vi "Compare Match Pattern.vi"(4 "use cached delimeter pattern data? (F)":bool, 6 "delimeters":cluster{"start":string, "end":string}={"start"="{{", "end"="}}"}, 7 "ignore case? (F)":bool, 8 "error in (no error)":errorcluster, 9 "substitutions":map{string, string}(c390), 11 "string to match":string) -> (0 "error out":errorcluster, 3 "match?":bool)   [LabVIEW 2019]
doc: "<b>Description</b> This VI applies compares a templated reference string against a map of replacements. Non-templated elements in the input string are ignored.\n\nFor example, if the string to match is \"{{Foo:bar}} {{Biz:BAZ}}\" and the map contains the definitions {Foo => bar, Biz: baz} and the ignore case input were TRUE, this VI would output match = TRUE.\n\n<b>Inputs</b>\n<b>substitutions</b>: A dictoinary of substitutions to apply to the input string.\n<b>delimeters</b>: The start and end delimeters for the desired substitution pattern. Defaults to '{{' and '}}'.\n<b>string to match</b>: A string containing substituions to match.\n\n<b>Outputs</b>\n<b>error out</b>: This VI will return error -1967345147 if a substitution key is missing from the input dictionary.\n<b>match?</b>: True if the template expression matches the contents of the map.\n\nBSD 3-Clause License\n\nCopyright (c) 2021, TauTerra, LLC\nAll rights reserved.\n\nRedistribution and use in source and binary forms, with or without\nmodification, are permitted provided that the following conditions are met:\n\n1. Redistributions of source code must retain the above copyright notice, this\n list of conditions and the following disclaimer.\n\n2. Redistributions in binary form must reproduce the above copyright notice,\n this list of conditions and the following disclaimer in the documentation\n and/or other materials provided with the distribution.\n\n3. Neither the name of the copyright holder nor the names of its\n contributors may be used to endorse or promote products derived from\n this software without specific prior written permission.\n\nTHIS SOFTWARE IS PROVIDED BY THE COPYRIGHT HOLDERS AND CONTRIBUTORS \"AS IS\"\nAND ANY EXPRESS OR IMPLIED WARRANTIES, INCLUDING, BUT NOT LIMITED TO, THE\nIMPLIED WARRANTIES OF MERCHANTABILITY AND FITNESS FOR A PARTICULAR PURPOSE ARE\nDISCLAIMED. IN NO EVENT SHALL THE COPYRIGHT HOLDER OR CONTRIBUTORS BE LIABLE\nFOR ANY DIRECT, INDIRECT, INCIDENTAL, SPECIAL, EXEMPLARY, OR CONSEQUENTIAL\nDAMAGES (INCLUDING, BUT NOT LIMITED TO, PROCUREMENT OF SUBSTITUTE GOODS OR\nSERVICES; LOSS OF USE, DATA, OR PROFITS; OR BUSINESS INTERRUPTION) HOWEVER\nCAUSED AND ON ANY THEORY OF LIABILITY, WHETHER IN CONTRACT, STRICT LIABILITY,\nOR TORT (INCLUDING NEGLIGENCE OR OTHERWISE) ARISING IN ANY WAY OUT OF THE USE\nOF THIS SOFTWARE, EVEN IF ADVISED OF THE POSSIBILITY OF SUCH DAMAGE."
uses:
  6811bf61-4d49-4179-8fc7-a72229c4be46.vi
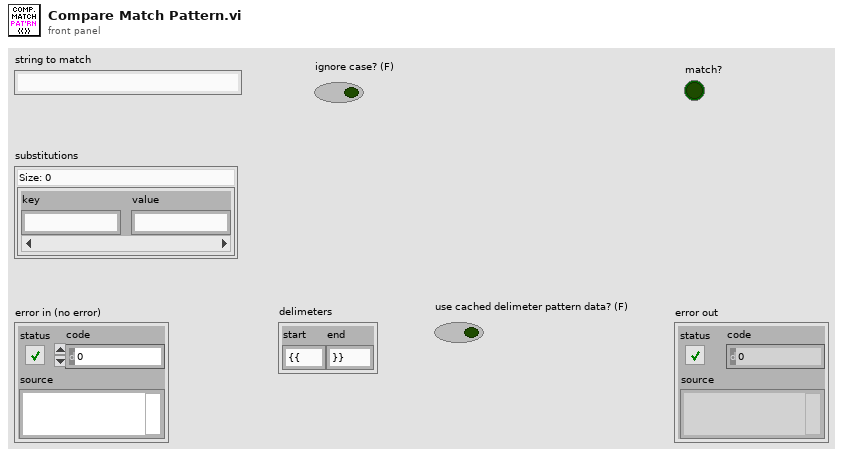
[diagram p1: front panel]
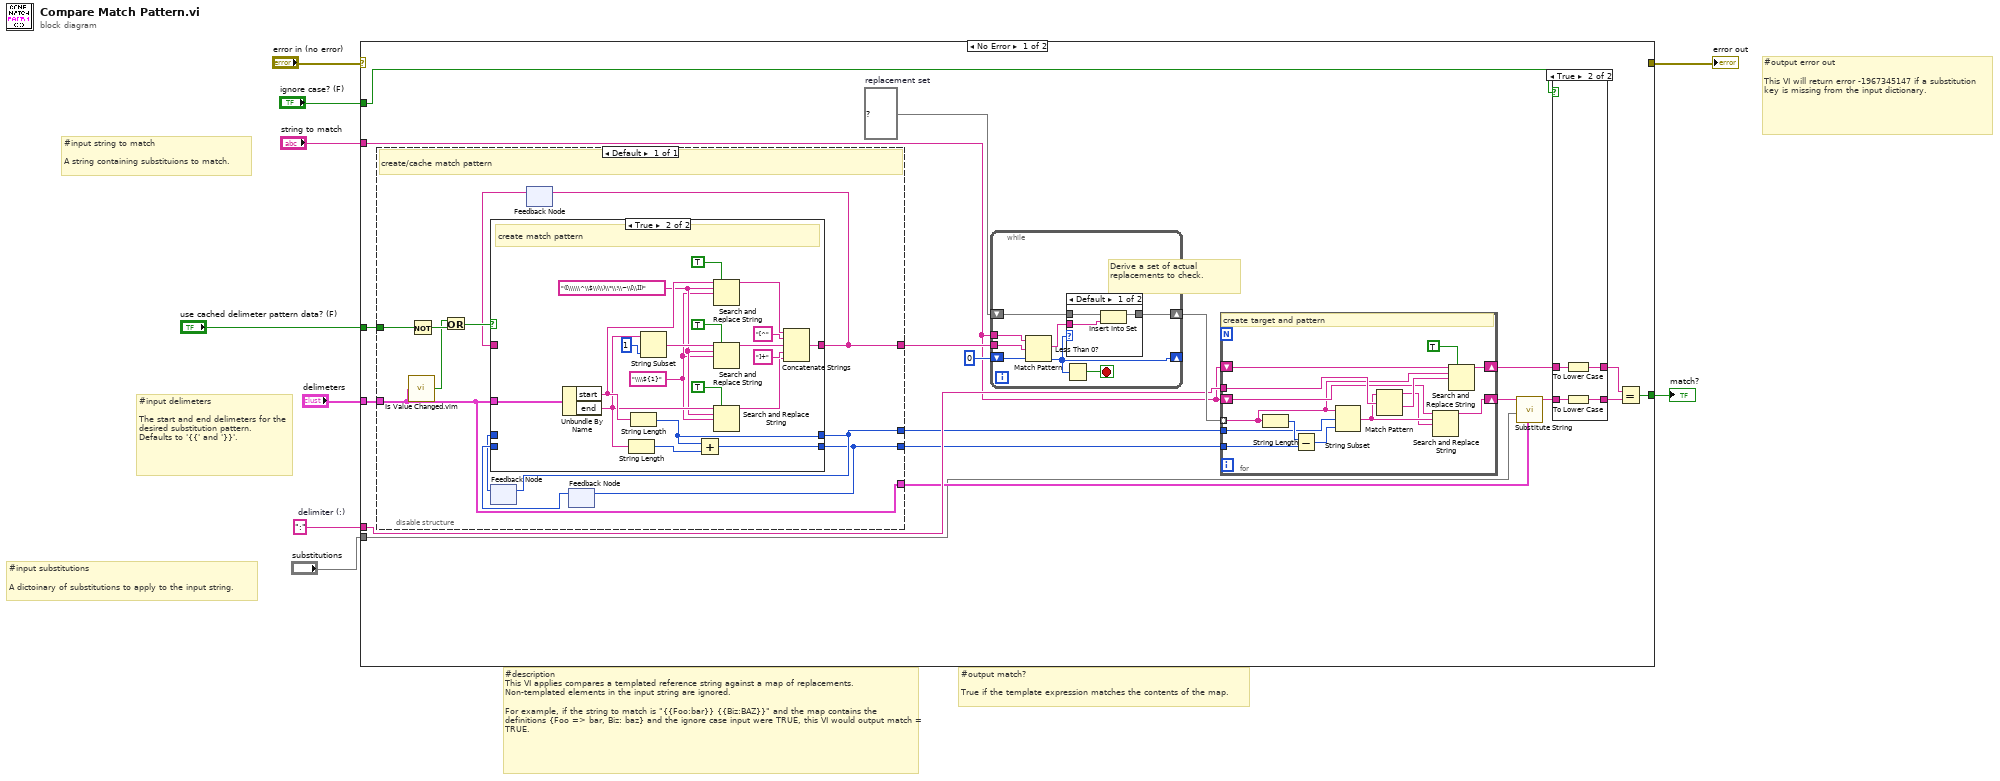
[diagram p0: block diagram]
diagram:
  w3 = ":"  # delimiter (:)
  # "#output error out\n\nThis VI will return error -1967345147 if a substitution key is missing from the input dictionary."
  # "#output match?\n\nTrue if the template expression matches the contents of the map."
  # "#input substitutions\n\nA dictoinary of substitutions to apply to the input string."
  # "#input delimeters\n\nThe start and end delimeters for the desired substitution pattern. Defaults to '{{' and '}}'."
  # "#input string to match\n\nA string containing substituions to match."
  # "#description\nThis VI applies compares a templated reference string against a map of replacements. Non-templated elements in the input string are ignored.\n\nFor example, if the string to match is \"{{Foo:bar}} {{Biz:BAZ}}\" and the map contains the definitions {Foo => bar, Biz: baz} and the ignore case input were TRUE, this VI would output match = TRUE."
  n1 = case shown="No Error" "error in (no error)" {
    selector: "error in (no error)" -> [_ w94]
    tunnel: "delimeters" -> [w26 _]
    tunnel: "string to match" -> [w19 _]
    tunnel: "substitutions" -> [w17 _]
    tunnel: [_ w94] -> w5
    tunnel: "use cached delimeter pattern data? (F)" -> [w25 _]
    tunnel: w3 -> [w22 _]
    tunnel: [w16 _] -> w2
    tunnel: "ignore case? (F)" -> [w15 _]
    frame No Error {
      w28 = set{string} {}  # replacement set
      n2 = disable-structure shown="Default" {
        disable-tunnel: w26 -> [w49]
        disable-tunnel: w25 -> [w59]
        disable-tunnel: [w55] -> w20
        disable-tunnel: [w54] -> w24
        disable-tunnel: [w53] -> w21
        disable-tunnel: [w49] -> w18
        frame Enabled {
          # "create/cache match pattern"
          n3 = call "Is Value Changed.vim"("value"=w49) -> ("changed or first call?"=w57:bool)
          n4 = Not(x=w59) -> (.not. x?=w58:bool)
          n5 = Or(x=w57, y=w58) -> (x .or. y?=w56:bool)
          n6 = feedback #1() -> (w50:i32)  [unwired: 1 in]
          n7 = feedback #2() -> (w51:string)  [unwired: 1 in]
          n8 = feedback #3() -> (w52:i32)  [unwired: 1 in]
          n9 = case shown="True" w56 {
            tunnel: [w61 w81] -> w54
            tunnel: [w62 w80] -> w53
            tunnel: [w60 w79] -> w55
            tunnel: w49 -> [_ w78]
            tunnel: w52 -> [w62 _]
            tunnel: w51 -> [w61 _]
            tunnel: w50 -> [w60 _]
            frame False {
            }
            frame True {
              w67 = "\\\\${1}" ("replace string (\"\")")
              w68 = "([\\\\\\^\\$\\(\\)\\*\\!\\~\\[\\]])" ("search string")
              # "create match pattern"
              n10 = Unbundle By Name(w78) -> ("start"=w75:string, "end"=w73:string)
              n11 = String Length(string=w73) -> (length=w74:i32)
              n12 = String Length(string=w75) -> (length=w79:i32)
              n13 = String Subset(string=w73, length (rest)=1 ("length (rest)")) -> (substring=w69:string)  [unwired: 1 in]
              n14 = Add(x=w79, y=w74) -> (x+y=w80:i32)
              n15 = Search and Replace String(replace all?=TRUE ("replace all? (F)"), input string=w75, search string=w68, replace string=w67) -> (result string=w77:string)  [unwired: 4 in, 3 out]
              n16 = Search and Replace String(replace all?=TRUE ("replace all? (F)"), input string=w69, search string=w68, replace string=w67) -> (result string=w65:string)  [unwired: 4 in, 3 out]
              n17 = Search and Replace String(replace all?=TRUE ("replace all? (F)"), input string=w73, search string=w68, replace string=w67) -> (result string=w63:string)  [unwired: 4 in, 3 out]
              n18 = Concatenate Strings(w77, "[^" ("string"), w65, "]+" ("string"), w63) -> (w81:string)
            }
          }
          n19 = feedback-in #1(w55) -> ()
          n20 = feedback-in #2(w54) -> ()
          n21 = feedback-in #3(w53) -> ()
        }
      }
      n22 = while {
        tunnel: w19 -> [w89]
        tunnel: w24 -> [w88]
        shift-right: [w84] -> w23
        shift-left: w28 -> [w85]
        shift-right: [w83] -> _
        shift-left: 0 ("offset past match") -> [w82]
        stop <- w87 stop-if-true
        # "Derive a set of actual replacements to check."
        n23 = Match Pattern(string=w89, regular expression=w88, offset (0)=w82) -> (match substring=w86:string, offset past match=w83:i32)  [unwired: 2 out]
        n24 = Less Than 0?(x=w83) -> (x < 0?=w87:bool)
        n25 = case shown="Default" w83 {
          tunnel: w86 -> [w90 _]
          tunnel: w85 -> [w92 w93]
          tunnel: [w91 w93] -> w84
          frame Default {
            n26 = Insert Into Set(10:w90, 11:w92) -> (3:w91:set{string})  [unwired: 1 out]
          }
          frame -1 {
          }
        }
      }
      n27 = for {
        tunnel: w23 -> [w38] mode=indexing
        shift-right: [w44] -> w14
        shift-left: w19 -> [w45]
        tunnel: w22 -> [w46]
        tunnel: w21 -> [w41]
        tunnel: w20 -> [w40]
        shift-right: [w35] -> w12
        shift-left: w19 -> [w39]
        # "create target and pattern"
        n28 = String Length(string=w38) -> (length=w48:i32)
        n29 = Subtract(x=w48, y=w41) -> (x-y=w47:i32)
        n30 = String Subset(string=w38, offset (0)=w40, length (rest)=w47) -> (substring=w37:string)
        n31 = Match Pattern(string=w37, regular expression=w46) -> (before substring=w36:string, after substring=w42:string)  [unwired: 1 in, 2 out]
        n32 = Search and Replace String(input string=w39, search string=w37, replace string=w36) -> (result string=w35:string)  [unwired: 5 in, 3 out]
        n33 = Search and Replace String(replace all?=TRUE ("replace all? (F)"), input string=w45, search string=w38, replace string=w42) -> (result string=w44:string)  [unwired: 4 in, 3 out]
      }
      n34 = call "Substitute String.vi"("delimeters"=w18, "substitutions"=w17, "input string"=w12) -> ("output string"=w11:string)  [unwired: 7 in, 1 out]
      n35 = case shown="True" w15 {
        tunnel: [w30 w33] -> w13
        tunnel: w14 -> [w30 w34]
        tunnel: [w29 w31] -> w10
        tunnel: w11 -> [w29 w32]
        frame False {
        }
        frame True {
          n36 = To Lower Case(string=w34) -> (all lower case string=w33:string)
          n37 = To Lower Case(string=w32) -> (all lower case string=w31:string)
        }
      }
      n38 = Equal?(x=w13, y=w10) -> (x = y?=w16:bool)
    }
    frame Error {
    }
  }
  "error out" <- w5
  "match?" <- w2
